vi "CustomerString.vi"(8 "error in (no error)":errorcluster, 10 "Shift String":string, 11 "unsigned byte array":u8[](array[numeric])) -> (0 "error out":errorcluster, 3 "String out":string)   [LabVIEW 2011]
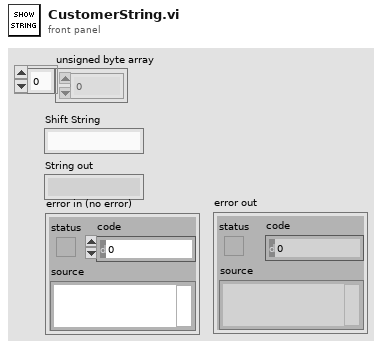
[diagram p1: front panel]
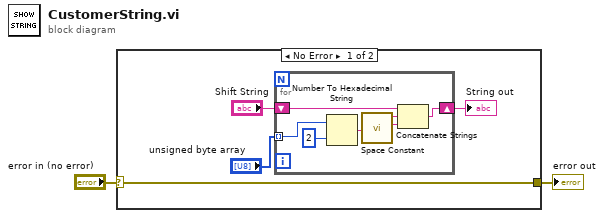
[diagram p0: block diagram]
diagram:
  n1 = case shown="No Error" "error in (no error)" {
    selector: "error in (no error)" -> [w3 w13]
    tunnel: [w3 w13] -> w1
    frame No Error {
      n2 = for {
        shift-right: [w11] -> w6
        shift-left: "Shift String" -> [w12]
        tunnel: "unsigned byte array" -> [w7] mode=indexing
        n3 = Number To Hexadecimal String(1:i16 2 ("width (-)"), 2:w7) -> (0:w10:string)
        n4 = call <vilib>:"Space Constant.vi"() -> ("String"=w9:string)
        n5 = Concatenate Strings(w12, w10, w9) -> (w11:string)
      }
      "String out" <- w6
    }
    frame Error {
    }
  }
  "error out" <- w1
